vi "Auto Adjust Shooter Angle.vi"() -> (2 "On Target":bool, 3 "zAvit Vbus Out":dbl)   [LabVIEW 2012]
uses:
  BotStatus.vi
  <vilib>/express/express arith-compare/Formula/XNode/ExpressFormulaBlockNode.xnode
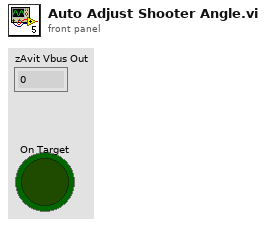
[diagram p1: front panel]
types:
  T1 = cluster{"Middle":bool, "InCannon":bool, "InFlipper":bool, "FlipperAtPlace":bool, "Bottom":bool, "FrisbeeDirection":bool}
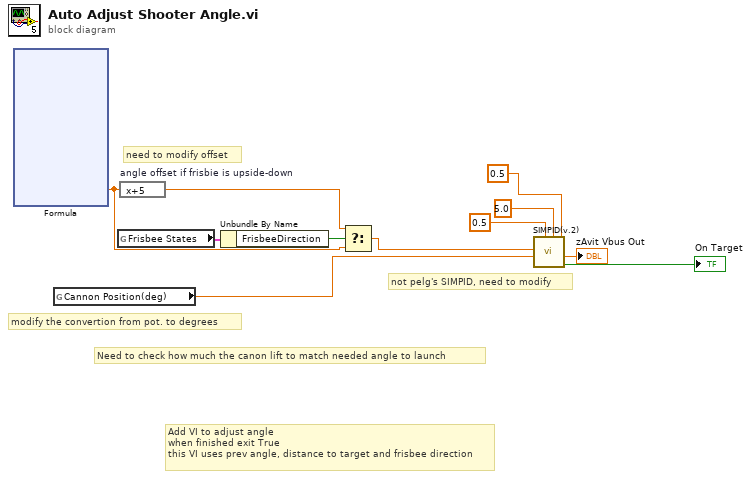
[diagram p0: block diagram]
diagram:
  # "not pelg's SIMPID, need to modify"
  # "Need to check how much the canon lift to match needed angle to launch"
  # "need to modify offset"
  # "modify the convertion from pot. to degrees"
  # "Add VI to adjust angle\nwhen finished exit True\nthis VI uses prev angle, distance to target and frisbee direction"
  n1 = xnode "Formula"() -> ("Result"=w8:dbl)  [unwired: 5 in, 1 out]
  n2 = global read "BotStatus.vi" "Cannon Position(deg)"() -> (w3:dbl)
  n3 = global read "BotStatus.vi" "Frisbee States"() -> (w10:T1)
  n4 = expression code="x+5" "angle offset if frisbie is upside-down"(w8) -> (w9:dbl)
  n5 = Unbundle By Name(w10) -> ("FrisbeeDirection"=w11:bool)
  n6 = Select(t=w9, s=w11, f=w8) -> (s? t:f=w4:dbl)
  n7 = call "SIMPID(v.2).vi"("Range"=0.5, "upper limit"=5.0, "lower limit"=0.5, "Current Point"=w3, "Set Point"=w4) -> ("On Target"=→"On Target":bool, "result"=→"zAvit Vbus Out":dbl)  [unwired: 5 in]
